vi "Datasheet Generate S#P.vi"(7 "System or ALL Combined Fields":T1[](array[typedef]), 8 "error in (no error)":errorcluster, 10 "Destination Directory (Temp)":path, 11 "File Information":T4) -> (0 "error out":errorcluster, 3 "SNP File Path":path)   [LabVIEW 2011]
uses:
  TDMS/TDMS File.ctl
  TDMS/TDMS Run.ctl
  TDMS/TDMS Channel (Sxx).ctl
  database/Fields/Field Record.ctl
  database/Fields/Field DataTypes.ctl
  database/Fields/Field NextItem.ctl
  Summitek EXT/OpenG EXT/array/array.llb/Sort 1D Array (String)__ogtk.vi
  Summitek EXT/OpenG EXT/array/array.llb/Reorder 1D Array2 (String)__ogtk.vi
panel:
  out "Concatenated String":string
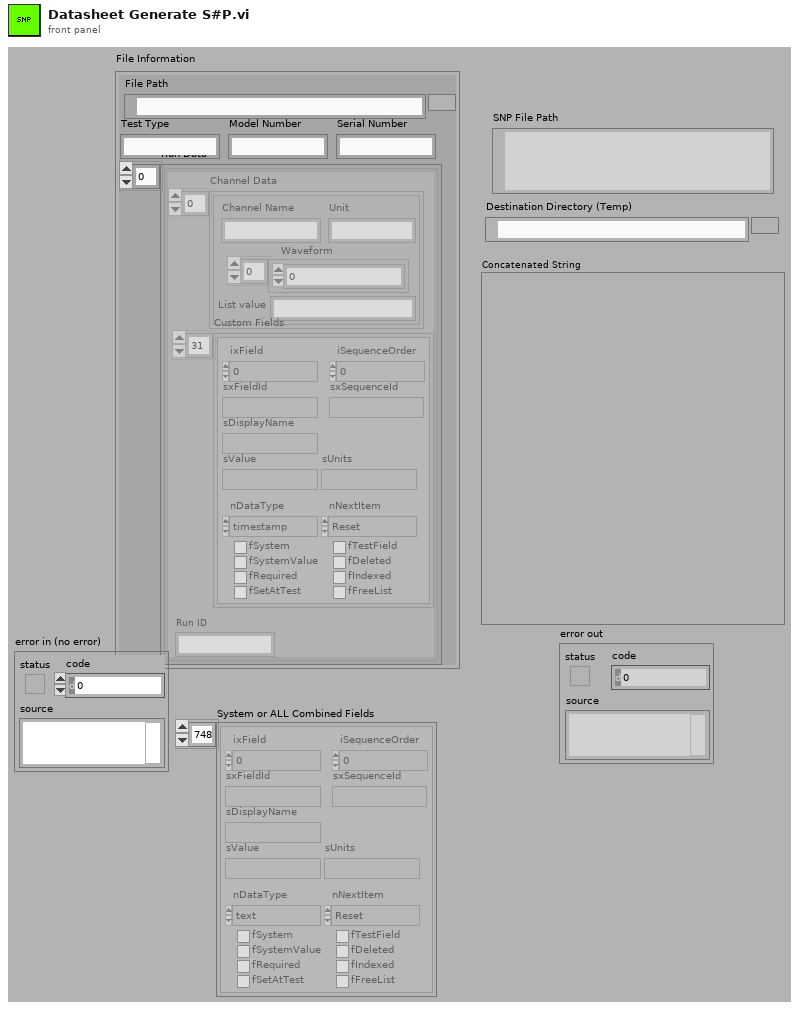
[diagram p1: front panel]
types:
  T1 = typedef "Field Record.ctl" = cluster{"ixField":i32, "iSequenceOrder":i32, "sxFieldId":string, "sxSequenceId":string, "sDisplayName":string, "sValue":string, "sUnits":string, "nDataType":T2, "nNextItem":T3, "fSystem":bool, "fSystemValue":bool, "fRequired":bool, "fSetAtTest":bool, "fTestField":bool, "fDeleted":bool, "fIndexed":bool, "fFreeList":bool}
  T2 = typedef "Field DataTypes.ctl" = enum32{"text", "numeric", "list", "timestamp", "boolean"}
  T3 = typedef "Field NextItem.ctl" = enum32{"Reset", "Retain", "Auto-Increment"}
  T4 = typedef "TDMS File.ctl" = cluster{"File Path":path, "Run Data":T5[], "Serial Number":string, "Model Number":string, "Test Type":string}
  T5 = typedef "TDMS Run.ctl" = cluster{"Channel Data":T6[], "Custom Fields":T1[], "Run ID":string}
  T6 = typedef "TDMS Channel (Sxx).ctl" = cluster{"Channel Name":string, "Waveform":dbl[], "Unit":string, "List value":string}
  T7 = enum16{"open", "replace", "create", "open or create", "replace or create", "replace or create with confirmation"}
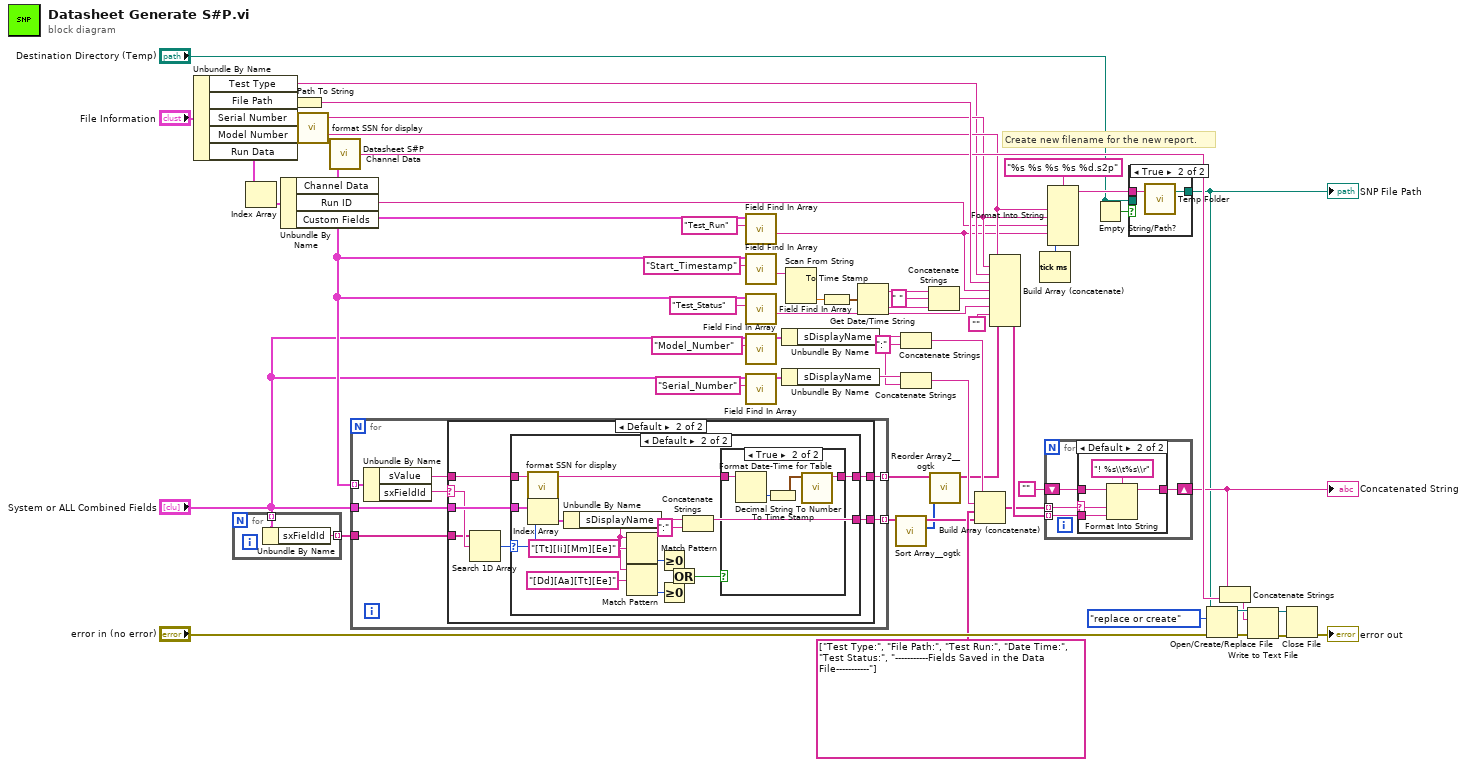
[diagram p0: block diagram]
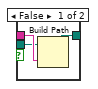
[diagram p2: hidden frame]
diagram:
  w6 = ":" ("string")
  # "Create new filename for the new report."
  n1 = Unbundle By Name("File Information") -> ("Test Type"=w17:string, "File Path"=w53:path, "Serial Number"=w45:string, "Model Number"=w19:string, "Run Data"=w60:T5[])
  n2 = for {
    tunnel: [w63] -> w32 mode=indexing
    tunnel: "System or ALL Combined Fields" -> [w62] mode=indexing
    n3 = Unbundle By Name(w62) -> ("sxFieldId"=w63:string)
  }
  n4 = Index Array(array=w60) -> (element=w24:T5)  [unwired: 1 in]
  n5 = Unbundle By Name(w24) -> ("Channel Data"=w22:T6[], "Run ID"=w13:string, "Custom Fields"=w28:T1[])
  n6 = Path To String(path=w53) -> (string=w52:string)
  n7 = call "format SSN for display.vi"("string"=w45) -> ("s? t:f"=w18:string)  [unwired: 4 out]
  n8 = call "Datasheet S#P Channel Data.vi"("Channel Data"=w22) -> ("HTM Table Rows"=w37:string)
  n9 = for {
    tunnel: w28 -> [w70] mode=indexing
    tunnel: [w68] -> w1 mode=indexing
    tunnel: "System or ALL Combined Fields" -> [w66]
    tunnel: [w67] -> w4 mode=indexing
    tunnel: w32 -> [w64]
    n10 = Unbundle By Name(w70) -> ("sValue"=w69:string, "sxFieldId"=w65:string)
    n11 = case shown="Default" w65 {
      selector: w65 -> [_ w72]
      tunnel: w69 -> [_ w77]
      tunnel: [_ w76] -> w68
      tunnel: [_ w75] -> w67
      tunnel: w66 -> [_ w74]
      tunnel: w64 -> [_ w71]
      frame "Model_Number", "Serial_Number", "Start_Timestamp", "Test_Run", "Test_Status", "Test_Type" {
      }
      frame Default {
        n12 = Search 1D Array(1D array=w71, element=w72) -> (index of element=w73:i32)  [unwired: 1 in]
        n13 = case shown="Default" w73 {
          selector: w73 -> [_ w90]
          tunnel: w77 -> [_ w93]
          tunnel: [_ w81] -> w76
          tunnel: [_ w78] -> w75
          tunnel: w74 -> [_ w92]
          frame -1 {
          }
          frame Default {
            n14 = call "format SSN for display.vi"("string"=w93) -> ("s? t:f"=w82:string)  [unwired: 4 out]
            n15 = Index Array(array=w92, index=w90) -> (element=w91:T1)
            n16 = Unbundle By Name(w91) -> ("sDisplayName"=w79:string)
            n17 = Match Pattern(string=w79, regular expression="[Tt][Ii][Mm][Ee]") -> (offset past match=w87:i32)  [unwired: 1 in, 3 out]
            n18 = Match Pattern(string=w79, regular expression="[Dd][Aa][Tt][Ee]") -> (offset past match=w86:i32)  [unwired: 1 in, 3 out]
            n19 = Greater Or Equal To 0?(x=w87) -> (x >= 0?=w85:bool)
            n20 = Greater Or Equal To 0?(x=w86) -> (x >= 0?=w84:bool)
            n21 = Or(x=w85, y=w84) -> (x .or. y?=w83:bool)
            n22 = Concatenate Strings(w79, ":" ("string")) -> (w78:string)
            n23 = case shown="True" w83 {
              tunnel: w82 -> [w94 w96]
              tunnel: [w94 w95] -> w81
              frame False {
              }
              frame True {
                n24 = Decimal String To Number(string=w96) -> (number=w98:i32)  [unwired: 2 in, 1 out]
                n25 = To Time Stamp(1:w98) -> (0:w97:timestamp)
                n26 = call "Format Date-Time for Table.vi"("Time Stamp"=w97) -> ("String"=w95:string)  [unwired: 10 in]
              }
            }
          }
        }
      }
    }
  }
  n27 = call "Field Find In Array.vi"("FieldID or Display Name(\"\")"="Test_Run" ("format string"), "Field Array"=w28) -> ("sValue"=w16:string)  [unwired: 1 in, 8 out]
  n28 = call "Field Find In Array.vi"("FieldID or Display Name(\"\")"="Start_Timestamp" ("format string"), "Field Array"=w28) -> ("sValue"=w39:string)  [unwired: 1 in, 8 out]
  n29 = call "Field Find In Array.vi"("FieldID or Display Name(\"\")"="Test_Status" ("format string"), "Field Array"=w28) -> ("sValue"=w38:string)  [unwired: 1 in, 8 out]
  n30 = call "Field Find In Array.vi"("FieldID or Display Name(\"\")"="Model_Number" ("format string"), "Field Array"="System or ALL Combined Fields") -> ("Field"=w27:T1)  [unwired: 1 in, 8 out]
  n31 = call "Field Find In Array.vi"("FieldID or Display Name(\"\")"="Serial_Number" ("format string"), "Field Array"="System or ALL Combined Fields") -> ("Field"=w26:T1)  [unwired: 1 in, 8 out]
  n32 = Unbundle By Name(w27) -> ("sDisplayName"=w10:string)
  n33 = Unbundle By Name(w26) -> ("sDisplayName"=w8:string)
  n34 = Scan From String(input string=w39) -> (output 1=w40:dbl)  [unwired: 3 in, 4 out]
  n35 = To Time Stamp(1:w40) -> (0:w41:timestamp)
  n36 = Get Date/Time String(seconds (now)=w41) -> (date string=w51:string, time string=w50:string)  [unwired: 2 out]
  n37 = call-poly "Sort Array__ogtk.vi"("Array in"=w4) -> ("Sorted Pointers"=w3:i32[], "Sorted Array out"=w5:string[])  [unwired: 9 in]
  n38 = Concatenate Strings(w10, w6) -> (w9:string)
  n39 = Concatenate Strings(w8, w6) -> (w7:string)
  n40 = Concatenate Strings(w51, " " ("regular expression"), w50) -> (w49:string)
  n41 = call-poly "Reorder Array2__ogtk.vi"("indices"=w3, "array"=w1) -> ("reordered array"=w2:string[])  [unwired: 9 in]
  n42 = Build Array (concatenate)(w9, w7, string[] ["Test Type:", "File Path:", "Test Run:", "Date Time:", "Test Status:", "-----------Fields Saved in the Data File-----------"], w5) -> (w47:string[])
  n43 = Build Array (concatenate)(w19, w18, w17, w52, w16, w49, w38, "" ("format string"), w2) -> (w48:string[])
  n44 = Tick Count (ms)() -> (millisecond timer value=w20:u32)
  n45 = for {
    shift-right: [w102] -> w35
    shift-left: "" -> [w101]
    tunnel: w48 -> [w100] mode=indexing
    tunnel: w47 -> [w99] mode=indexing
    n46 = case shown="Default" w99 {
      selector: w99 -> [_ w104]
      tunnel: [w103 w107] -> w102
      tunnel: w101 -> [w103 w106]
      tunnel: w100 -> [_ w105]
      frame "" {
      }
      frame Default {
        n47 = Format Into String(format string="! %s\\t%s\\r", initial string=w106, w104, w105) -> (resulting string=w107:string)  [unwired: 1 in, 1 out]
      }
    }
  }
  "Concatenated String" <- w35
  n48 = Format Into String(format string="%s %s %s %s %d.s2p", w19, w18, w13, w16, w20) -> (resulting string=w15:string)  [unwired: 2 in, 1 out]
  n49 = Empty String/Path?(string/path="Destination Directory (Temp)") -> (empty?=w12:bool)
  n50 = case shown="True" w12 {
    tunnel: [w111 w113] -> w33
    tunnel: w15 -> [w110 w112]
    tunnel: "Destination Directory (Temp)" -> [w109 _]
    frame False {
      n51 = Build Path(base path=w109, name or relative path=w110) -> (appended path=w111:path)
    }
    frame True {
      n52 = call "Temp Folder.vi"("Relative Path (\"\")"=w112) -> ("Temp Folder"=w113:path)  [unwired: 2 in]
    }
  }
  "SNP File Path" <- w33
  n53 = Open/Create/Replace File(file path (use dialog)=w33, error in="error in (no error)", operation (0:open)=T7."replace or create") -> (refnum out=w58:refnum<file>, error out=w57:errorcluster)  [unwired: 4 out]
  n54 = Concatenate Strings(w35, w37) -> (w36:string)
  n55 = Write to Text File(file (use dialog)=w58, text=w36, error in=w57) -> (refnum out=w56:refnum<file>, error out=w55:errorcluster)  [unwired: 2 out]
  n56 = Close File(refnum=w56, error in=w55) -> (error out=→"error out":errorcluster)  [unwired: 1 out]
